vi "Configure Fast Acquisition.vi"(8 "error in (no error)":errorcluster, 9 "Enable Fast Acquisition (F: Disable)":bool, 10 "Waveform Grading (1: Temperature)":i32(ring)=1 items=["Normal", "Temperature", "Spectral", "Inverted"], 11 "VISA resource name":refnum<visa-resource-name>) -> (0 "error out":errorcluster, 3 "VISA resource name out":refnum<visa-resource-name>)   [LabVIEW 2017, in "Scope.lvlib" / "Tektronix DPO MSO 2000 4000 Series.lvlib"]
doc: "Configures the fast acquisition mode.\n\n<B>Notes:</B>\n(1) This VI is available for MDO3000 Series only.\n\n(2) In fast acquisition mode, waveforms cannot be queried, saved or recalled, and reference waveforms cannot be turned on."
uses:
  Tektronix DPO MSO 2000 4000 Series.lvlib
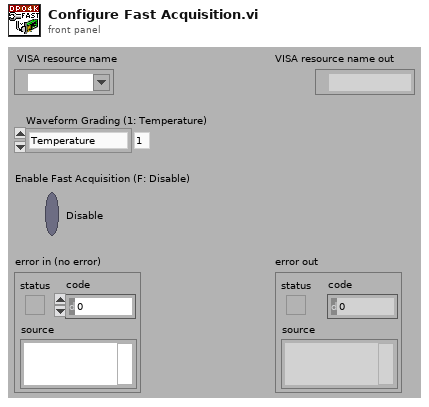
[diagram p1: front panel]
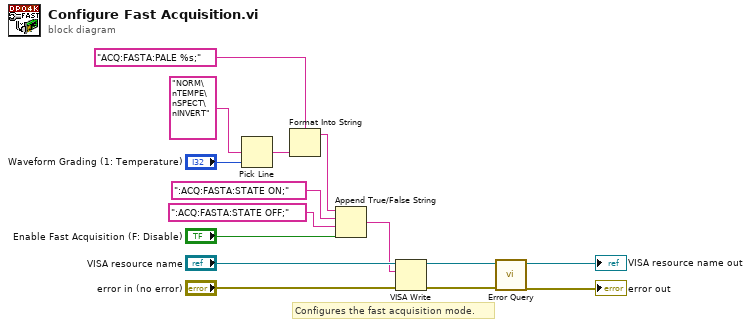
[diagram p0: block diagram]
diagram:
  # "Configures the fast acquisition mode."
  n1 = Pick Line(multi-line string="NORM\nTEMPE\nSPECT\nINVERT", line index="Waveform Grading (1: Temperature)") -> (output string=w3:string)  [unwired: 1 in]
  n2 = Format Into String(format string="ACQ:FASTA:PALE %s;", w3) -> (resulting string=w1:string)  [unwired: 2 in, 1 out]
  n3 = Append True/False String(1:"Enable Fast Acquisition (F: Disable)", 2:":ACQ:FASTA:STATE OFF;", 3:":ACQ:FASTA:STATE ON;", 4:w1) -> (0:w4:string)
  n4 = VISA Write(VISA resource name="VISA resource name", write buffer=w4, error in (no error)="error in (no error)") -> (VISA resource name out=w11:refnum<visa-resource-name>, error out=w10:errorcluster)  [unwired: 1 out]
  n5 = call "Error Query.vi"("error in (no error)"=w10, "VISA resource name"=w11) -> ("error out"=→"error out":errorcluster, "VISA resource name out"=→"VISA resource name out":refnum<visa-resource-name>)  [unwired: 6 in, 2 out]
